vi "Main.vi"() -> ()   [LabVIEW 2023]
uses:
  <userlib>/_OpenG.lib/array/array.llb/Empty 1D Array (DBL)__ogtk.vi
  <userlib>/_OpenG.lib/array/array.llb/openg_array.lvlib
panel:
  out "Empty Array?":bool
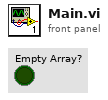
[diagram p1: front panel]
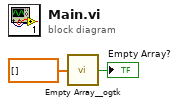
[diagram p0: block diagram]
diagram:
  n1 = call-poly <userlib>:"Empty Array__ogtk.vi"("Array"=dbl[] []) -> ("Empty Array?"=→"Empty Array?":bool)  [unwired: 8 in]
